vi "Software Update HCC Find Selected Stations.vi"(8 "Error In":errorcluster, 10 "Active Stations with Board IDs":string[][](array[string]), 11 "Update Files (Option 1-24)":i32[](array[numeric])) -> (0 "Error Out":errorcluster, 2 "Station Labels":string[](array[string]), 3 "Selected Board Indexes":i32[](array[numeric]))   [LabVIEW 2014]
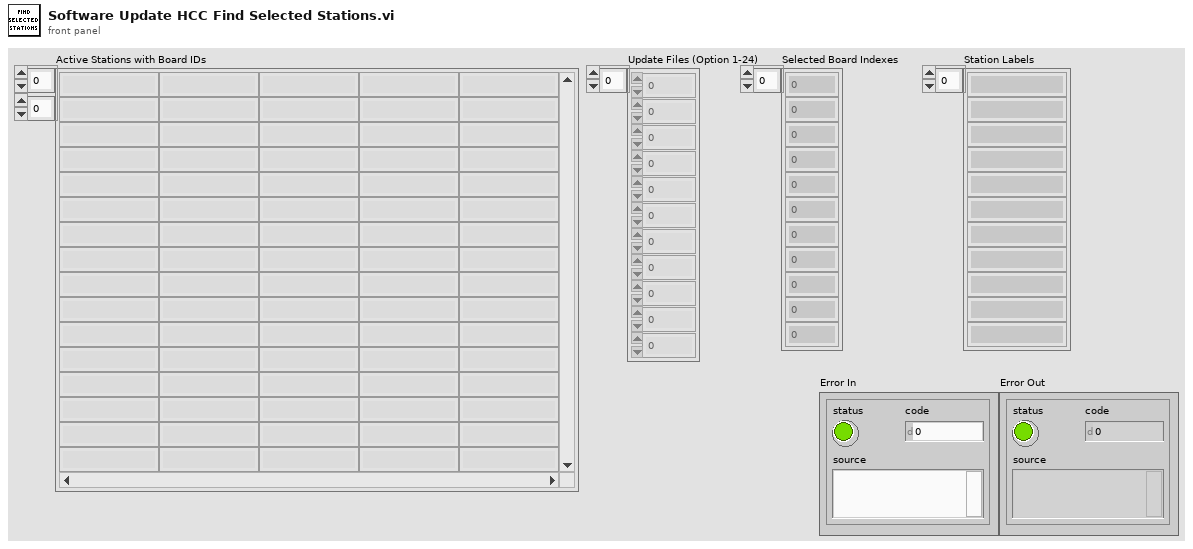
[diagram p1: front panel]
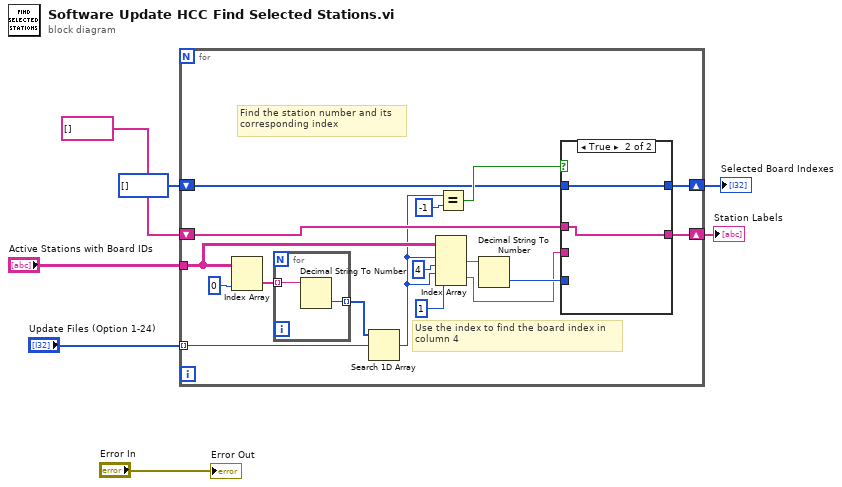
[diagram p0: block diagram]
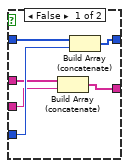
[diagram p2: hidden frame]
diagram:
  n1 = for {
    tunnel: "Active Stations with Board IDs" -> [w16]
    tunnel: "Update Files (Option 1-24)" -> [w17] mode=indexing
    shift-right: [w18] -> w5
    shift-left: i32[] [] -> [w19]
    shift-right: [w11] -> w1
    shift-left: string[] [] -> [w12]
    # "Use the index to find the board index in\ncolumn 4"
    # "Find the station number and its\ncorresponding index"
    n2 = Index Array(array=w16, index (col)=0 ("index")) -> (element=w23:string[])  [unwired: 1 in]
    n3 = for {
      tunnel: w23 -> [w34] mode=indexing
      tunnel: [w33] -> w22 mode=indexing
      n4 = Decimal String To Number(string=w34) -> (number=w33:i32)  [unwired: 2 in, 1 out]
    }
    n5 = Search 1D Array(1D array=w22, element=w17) -> (index of element=w10:i32)  [unwired: 1 in]
    n6 = Index Array(array=w16, index (row) #1=w10, index (col) #1=4 ("disabled index (col)"), index (row) #2=w10, index (col) #2=1 ("disabled index (col)")) -> (element #1=w14:string, element #2=w8:string)
    n7 = Equal?(x=w10, y=-1) -> (x = y?=w20:bool)
    n8 = Decimal String To Number(string=w14) -> (number=w13:i32)  [unwired: 2 in, 1 out]
    n9 = case shown="True" w20 {
      tunnel: w19 -> [w30 w32]
      tunnel: [w28 w32] -> w18
      tunnel: w13 -> [w29 _]
      tunnel: w12 -> [w27 w31]
      tunnel: [w26 w31] -> w11
      tunnel: w8 -> [w25 _]
      frame False {
        n10 = Build Array (concatenate)(w27, w25) -> (w26:string[])
        n11 = Build Array (concatenate)(w30, w29) -> (w28:i32[])
      }
      frame True {
      }
    }
  }
  "Selected Board Indexes" <- w5
  "Station Labels" <- w1
  "Error Out" <- "Error In"
